vi "Manager QueryPlugin.vi"(6 "contextId":T1, 8 "error in":errorcluster, 9 "timeout (ms)":i32=-1, 10 "Request Data":T15, 11 "gRPC ID":T1) -> (0 "error out":errorcluster, 2 "Response Data":T2, 3 "gRPC ID out":T1)   [LabVIEW 2021, in "CIF_Manager_client.lvlib"]
uses:
  CIF_Manager_client.lvlib
  <vilib>/gRPC/LabVIEW gRPC Library/Shared/grpcId.ctl
  RPC Messages/cif_manager_PluginName.ctl
  RPC Messages/cif_manager_PluginInfoResponse.ctl
  RPC Messages/cif_manager_PluginInfo.ctl
  RPC Messages/cif_manager_PluginVersion.ctl
  RPC Messages/cif_plugincore_StatusData.ctl
  RPC Messages/cif_plugincore_StatusData_State.ctl
  RPC Messages/cif_plugincore_TimingStatistics.ctl
  RPC Messages/cif_plugincore_TimingStatsBasic.ctl
  RPC Messages/cif_plugincore_FifoStatistics.ctl
  RPC Messages/cif_plugincore_Error.ctl
  RPC Messages/cif_plugincore_MonitorDoubles.ctl
  RPC Messages/cif_plugincore_MonitorU64.ctl
  RPC Messages/cif_plugincore_MonitorI64.ctl
  RPC Messages/cif_manager_Error.ctl
  RPC Messages/cif_manager_PluginInfoResponse_Flat.ctl
  RPC Messages/cif_manager_PluginInfo_Flat.ctl
  RPC Messages/cif_manager_PluginVersion_Flat.ctl
  RPC Messages/cif_plugincore_StatusData_Flat.ctl
  RPC Messages/cif_plugincore_TimingStatistics_Flat.ctl
  RPC Messages/cif_plugincore_TimingStatsBasic_Flat.ctl
  RPC Messages/cif_plugincore_FifoStatistics_Flat.ctl
  RPC Messages/cif_plugincore_Error_Flat.ctl
  RPC Messages/cif_plugincore_MonitorDoubles_Flat.ctl
  RPC Messages/cif_plugincore_MonitorU64_Flat.ctl
  RPC Messages/cif_plugincore_MonitorI64_Flat.ctl
  RPC Messages/cif_manager_Error_Flat.ctl
  14035477-4c25-4107-8ed5-d0c4ef420ce5.vi
  <vilib>/gRPC/LabVIEW gRPC Library/Shared/TranslateGrpcError.vi
  <vilib>/gRPC/LabVIEW gRPC Library/Shared/Wait On Occurrence Wrapper.vi
  RPC Messages/FlatToRichcif_manager_PluginInfo.vi
  RPC Messages/FlatToRichcif_manager_Error.vi
  <vilib>/gRPC/LabVIEW gRPC Library/Shared/Wait On Occurence.vi
  RPC Messages/FlatToRichcif_manager_PluginVersion.vi
  RPC Messages/FlatToRichcif_plugincore_StatusData.vi
  RPC Messages/FlatToRichcif_plugincore_TimingStatistics.vi
  RPC Messages/FlatToRichcif_plugincore_FifoStatistics.vi
  RPC Messages/FlatToRichcif_plugincore_Error.vi
  RPC Messages/FlatToRichcif_plugincore_MonitorDoubles.vi
  RPC Messages/FlatToRichcif_plugincore_MonitorU64.vi
  RPC Messages/FlatToRichcif_plugincore_MonitorI64.vi
  RPC Messages/FlatToRichcif_plugincore_TimingStatsBasic.vi
  <vilib>/gRPC/LabVIEW gRPC Library/Server API/Server/Get Server DLL Path.vi
  <vilib>/Utility/error.llb/Error Cluster From Error Code.vi
  <vilib>/Utility/config.llb/Open Config Data.vi
  <vilib>/Utility/config.llb/Write Key.vi
  <vilib>/Utility/config.llb/Write Key (Boolean).vi
  <vilib>/Utility/config.llb/Not A Config Data Refnum.vi
  <vilib>/Utility/config.llb/Read Key.vi
  <vilib>/Utility/config.llb/Read Key (Boolean).vi
  <vilib>/Utility/config.llb/Close Config Data.vi
  <vilib>/gRPC/LabVIEW gRPC Library/grpc-lvsupport-release.lvlib
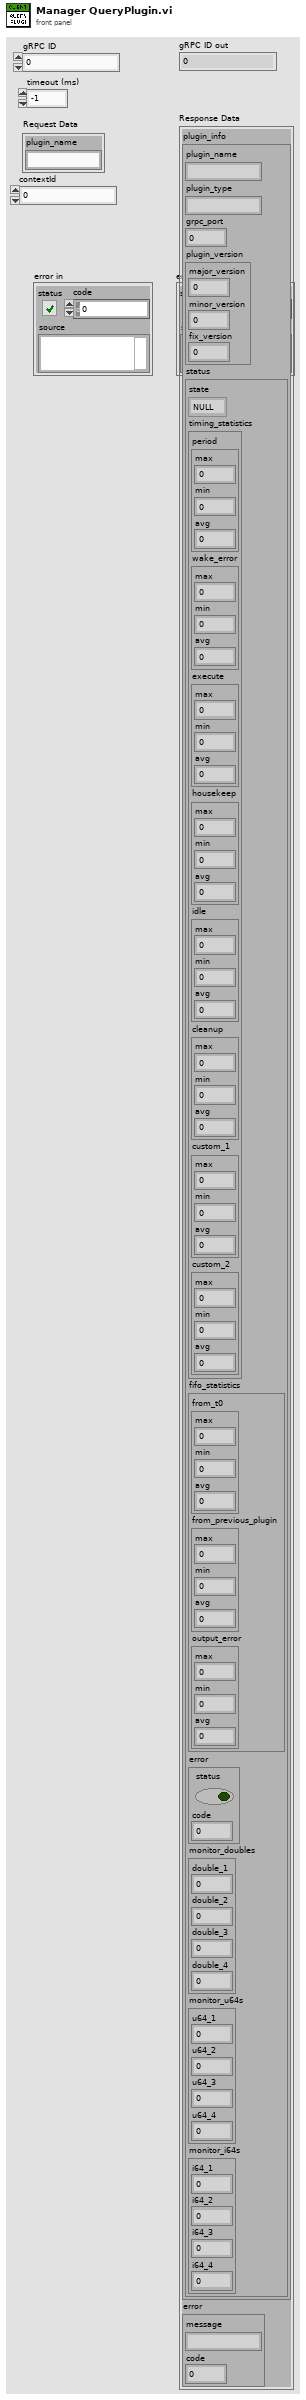
[diagram p1: front panel]
types:
  T1 = typedef "grpc-lvsupport-release.lvlib/grpcId.ctl" = u64
  T2 = typedef "CIF_Manager_client.lvlib/cif_manager_PluginInfoResponse.ctl" = cluster{"plugin_info":T3, "error":T14}
  T3 = typedef "CIF_Manager_client.lvlib/cif_manager_PluginInfo.ctl" = cluster{"plugin_name":string, "plugin_type":string, "grpc_port":i32, "plugin_version":T4, "status":T5}
  T4 = typedef "CIF_Manager_client.lvlib/cif_manager_PluginVersion.ctl" = cluster{"major_version":i32, "minor_version":i32, "fix_version":i32}
  T5 = typedef "CIF_Manager_client.lvlib/cif_plugincore_StatusData.ctl" = cluster{"state":T6, "timing_statistics":T7, "fifo_statistics":T9, "error":T10, "monitor_doubles":T11, "monitor_u64s":T12, "monitor_i64s":T13}
  T6 = typedef "CIF_Manager_client.lvlib/cif_plugincore_StatusData_State.ctl" = enum32{"NULL", "CREATING", "LISTENING", "RUNNING", "CLEANINGUP", "DESTROYING"}
  T7 = typedef "CIF_Manager_client.lvlib/cif_plugincore_TimingStatistics.ctl" = cluster{"period":T8, "wake_error":T8, "execute":T8, "housekeep":T8, "idle":T8, "cleanup":T8, "custom_1":T8, "custom_2":T8}
  T8 = typedef "CIF_Manager_client.lvlib/cif_plugincore_TimingStatsBasic.ctl" = cluster{"max":i64, "min":i64, "avg":dbl}
  T9 = typedef "CIF_Manager_client.lvlib/cif_plugincore_FifoStatistics.ctl" = cluster{"from_t0":T8, "from_previous_plugin":T8, "output_error":T8}
  T10 = typedef "CIF_Manager_client.lvlib/cif_plugincore_Error.ctl" = cluster{"status":bool, "code":i32}
  T11 = typedef "CIF_Manager_client.lvlib/cif_plugincore_MonitorDoubles.ctl" = cluster{"double_1":dbl, "double_2":dbl, "double_3":dbl, "double_4":dbl}
  T12 = typedef "CIF_Manager_client.lvlib/cif_plugincore_MonitorU64.ctl" = cluster{"u64_1":u64, "u64_2":u64, "u64_3":u64, "u64_4":u64}
  T13 = typedef "CIF_Manager_client.lvlib/cif_plugincore_MonitorI64.ctl" = cluster{"i64_1":i64, "i64_2":i64, "i64_3":i64, "i64_4":i64}
  T14 = typedef "CIF_Manager_client.lvlib/cif_manager_Error.ctl" = cluster{"message":string, "code":i32}
  T15 = typedef "CIF_Manager_client.lvlib/cif_manager_PluginName.ctl" = cluster{"plugin_name":string}
  T16 = typedef "CIF_Manager_client.lvlib/cif_manager_PluginInfoResponse_Flat.ctl" = cluster{"plugin_info":T17, "error":T27}
  T17 = typedef "CIF_Manager_client.lvlib/cif_manager_PluginInfo_Flat.ctl" = cluster{"plugin_name":string, "plugin_type":string, "grpc_port":i32, "plugin_version":T18, "status":T19}
  T18 = typedef "CIF_Manager_client.lvlib/cif_manager_PluginVersion_Flat.ctl" = cluster{"major_version":i32, "minor_version":i32, "fix_version":i32}
  T19 = typedef "CIF_Manager_client.lvlib/cif_plugincore_StatusData_Flat.ctl" = cluster{"state":T6, "timing_statistics":T20, "fifo_statistics":T22, "error":T23, "monitor_doubles":T24, "monitor_u64s":T25, "monitor_i64s":T26}
  T20 = typedef "CIF_Manager_client.lvlib/cif_plugincore_TimingStatistics_Flat.ctl" = cluster{"period":T21, "wake_error":T21, "execute":T21, "housekeep":T21, "idle":T21, "cleanup":T21, "custom_1":T21, "custom_2":T21}
  T21 = typedef "CIF_Manager_client.lvlib/cif_plugincore_TimingStatsBasic_Flat.ctl" = cluster{"max":i64, "min":i64, "avg":dbl}
  T22 = typedef "CIF_Manager_client.lvlib/cif_plugincore_FifoStatistics_Flat.ctl" = cluster{"from_t0":T21, "from_previous_plugin":T21, "output_error":T21}
  T23 = typedef "CIF_Manager_client.lvlib/cif_plugincore_Error_Flat.ctl" = cluster{"status":bool, "code":i32}
  T24 = typedef "CIF_Manager_client.lvlib/cif_plugincore_MonitorDoubles_Flat.ctl" = cluster{"double_1":dbl, "double_2":dbl, "double_3":dbl, "double_4":dbl}
  T25 = typedef "CIF_Manager_client.lvlib/cif_plugincore_MonitorU64_Flat.ctl" = cluster{"u64_1":u64, "u64_2":u64, "u64_3":u64, "u64_4":u64}
  T26 = typedef "CIF_Manager_client.lvlib/cif_plugincore_MonitorI64_Flat.ctl" = cluster{"i64_1":i64, "i64_2":i64, "i64_3":i64, "i64_4":i64}
  T27 = typedef "CIF_Manager_client.lvlib/cif_manager_Error_Flat.ctl" = cluster{"message":string, "code":i32}
  T28 = typedef "CIF_Manager_client.lvlib/cif_manager_PluginName_Flat.ctl" = cluster{"plugin_name":string}
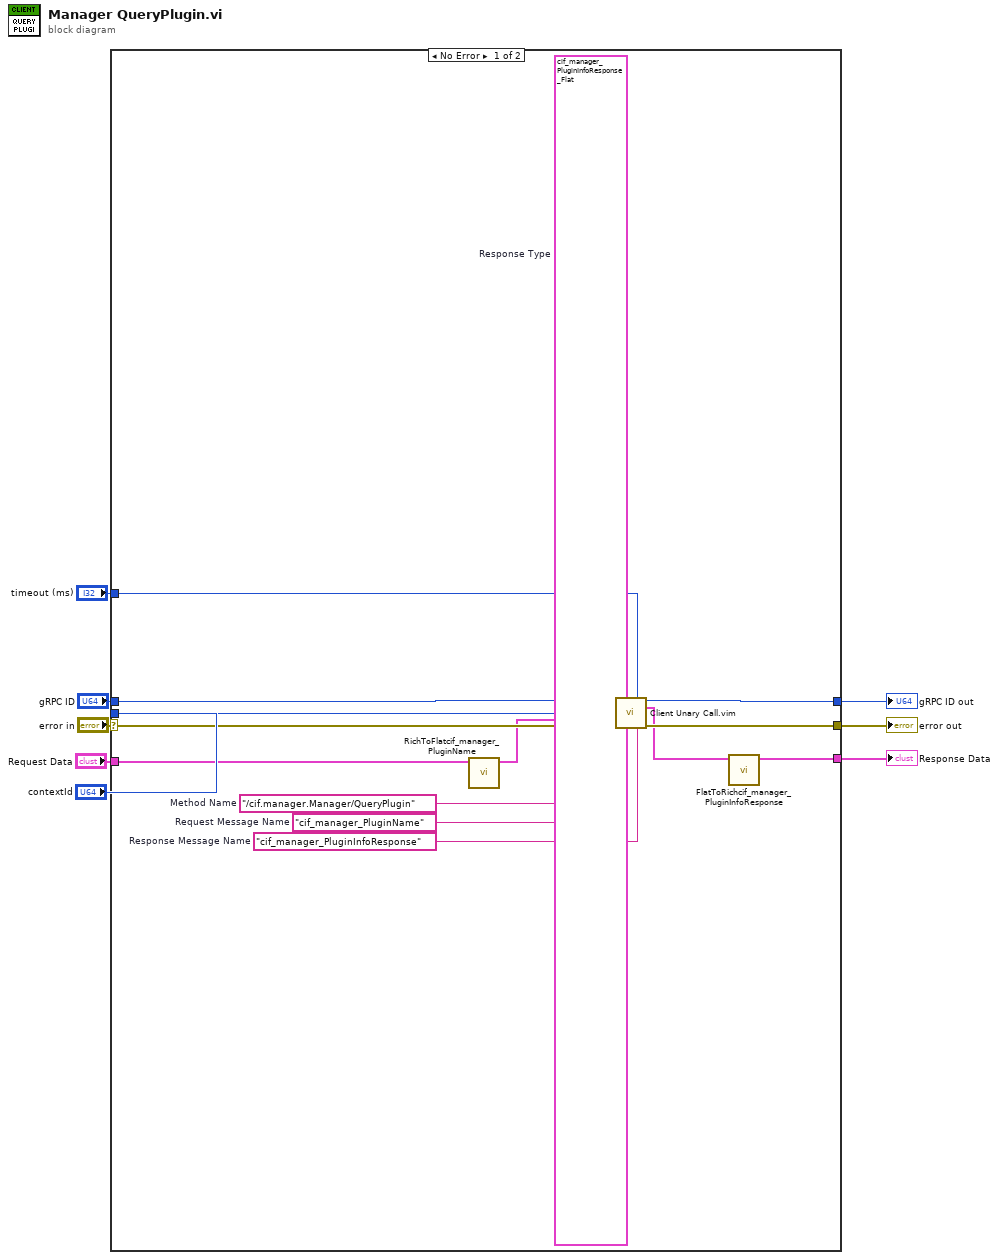
[diagram p0: block diagram]
diagram:
  n1 = case shown="No Error" "error in" {
    selector: "error in" -> [w18 w23]
    tunnel: [w17 w23] -> w7
    tunnel: "gRPC ID" -> [w16 w24]
    tunnel: [w15 w24] -> w5
    tunnel: "Request Data" -> [w12 _]
    tunnel: [w9 _] -> w3
    tunnel: "timeout (ms)" -> [w14 _]
    tunnel: "contextId" -> [w13 _]
    frame No Error {
      w19 = "cif_manager_PluginInfoResponse"  # Response Message Name
      w20 = "cif_manager_PluginName"  # Request Message Name
      w21 = T16 {"plugin_info"={"plugin_name"="", "plugin_type"="", "grpc_port"=0, "plugin_version"={"major_version"=0, "minor_version"=0, "fix_version"=0}, "status"={"state"=enum."NULL", "timing_statistics"={"period"={"max"=0, "min"=0, "avg"=0.0}, "wake_error"={"max"=0, "min"=0, "avg"=0.0}, "execute"={"max"=0, "min"=0, "avg"=0.0}, "housekeep"={"max"=0, "min"=0, "avg"=0.0}, "idle"={"max"=0, "min"=0, "avg"=0.0}, "cleanup"={"max"=0, "min"=0, "avg"=0.0}, "custom_1"={"max"=0, "min"=0, "avg"=0.0}, "custom_2"={"max"=0, "min"=0, "avg"=0.0}}, "fifo_statistics"={"from_t0"={"max"=0, "min"=0, "avg"=0.0}, "from_previous_plugin"={"max"=0, "min"=0, "avg"=0.0}, "output_error"={"max"=0, "min"=0, "avg"=0.0}}, "error"={"status"=FALSE, "code"=0}, "monitor_doubles"={"double_1"=0.0, "double_2"=0.0, "double_3"=0.0, "double_4"=0.0}, "monitor_u64s"={"u64_1"=0, "u64_2"=0, "u64_3"=0, "u64_4"=0}, "monitor_i64s"={"i64_1"=0, "i64_2"=0, "i64_3"=0, "i64_4"=0}}}, "error"={"message"="", "code"=0}}  # Response Type
      w22 = "/cif.manager.Manager/QueryPlugin"  # Method Name
      n2 = call "RichToFlatcif_manager_PluginName.vi"("InputCluster"=w12) -> ("OutputCluster"=w11:T28)  [unwired: 10 in]
      n3 = call "Client Unary Call.vim"("ClientID in"=w16, "Response Type"=w21, "timeout (ms)"=w14, "Method Name"=w22, "contextId"=w13, "Request Data"=w11, "error in"=w18, "Request Message Name"=w20, "Response Message Name"=w19) -> ("ClientID out"=w15:u64, "Response Data"=w10:T16, "error out"=w17:errorcluster)  [unwired: 4 in]
      n4 = call "FlatToRichcif_manager_PluginInfoResponse.vi"("InputCluster"=w10) -> ("OutputCluster"=w9:T2)  [unwired: 10 in]
    }
    frame Error {
    }
  }
  "error out" <- w7
  "gRPC ID out" <- w5
  "Response Data" <- w3
